vi "Rotate to Scrollback.vi"(7 "Scrollback":refnum<class "TermBuffer.lvclass">, 8 "error in (no error)":errorcluster, 11 "TermBuffer in":refnum<class "TermBuffer.lvclass">) -> (0 "error out":errorcluster, 3 "TermBuffer out":refnum<class "TermBuffer.lvclass">)   [LabVIEW 2020, in "Terminal.lvlib" / "TermBuffer.lvclass"]
uses:
  TermBuffer.lvclass
  TermBuffer.lvclass/TermBuffer.ctl
  TermLine/TermLine.lvclass
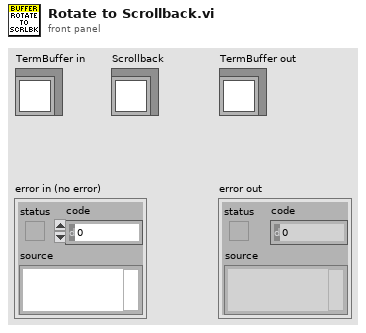
[diagram p1: front panel]
types:
  T1 = typedef "Terminal.lvlib/TermBuffer.lvclass/Ref Data.ctl" = cluster{"Lines":refnum<class "TermLine.lvclass">[], "Rows":i32, "Cols":i32}
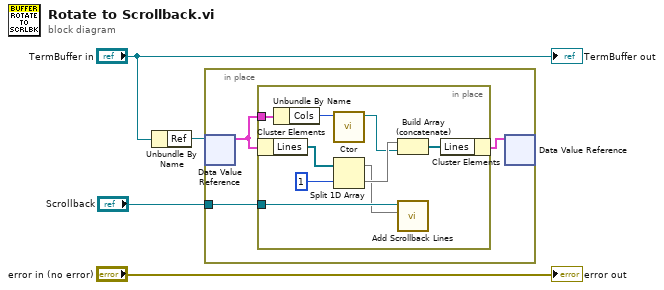
[diagram p0: block diagram]
diagram:
  n1 = Unbundle By Name("TermBuffer in") -> ("Ref"=w3:refnum<data-value>)
  n2 = in-place {
    in-place-border: "Scrollback" -> [w5]
    n3 = in-place-dvr #1(w3) -> (w6:T1)  [unwired: 1 out]
    n4 = in-place {
      in-place-border: w6 -> [w11]
      in-place-border: w5 -> [w9]
      n5 = in-place-cluster #2(w6) -> ("Lines"=w16:refnum<class "TermLine.lvclass">[])
      n6 = Unbundle By Name(w11) -> ("Cols"=w10:i32)
      n7 = call "Ctor.vi"("Width (0)"=w10) -> ("TermLine out"=w12:refnum<class "TermLine.lvclass">)  [unwired: 9 in, 1 out]
      n8 = Split 1D Array(array=w16, index=1) -> (first subarray=w8:refnum<class "TermLine.lvclass">[], second subarray=w14:refnum<class "TermLine.lvclass">[])
      n9 = Build Array (concatenate)(w14, w12) -> (w13:refnum<class "TermLine.lvclass">[])
      n10 = call "Add Scrollback Lines.vi"("Lines"=w8, "TermBuffer in"=w9) -> ()  [unwired: 8 in, 2 out]
      n11 = in-place-cluster #2("Lines"=w13) -> (w7:T1)
    }
    n12 = in-place-dvr #1(w7) -> ()  [unwired: 2 out]
  }
  "error out" <- "error in (no error)"
  "TermBuffer out" <- "TermBuffer in"
